vi "continous_to_binary.vi"() -> ()   [LabVIEW 2018]
uses:
  <vilib>/measure/NI_MABase.lvlib
panel:
  out "Waveform Graph 5":waveform(dbl)(graph)
  out "Waveform Graph 3":waveform(dbl)(graph)
  out "size(s)":i32
  out "Waveform Graph 2":waveform(dbl)(graph)
  in  "Fréquence":dbl(knob)=10.988369287950603 scale=0.0..100.0
  in  "Amplitude":dbl(knob)=1.3927187800734715 scale=0.0..10.0
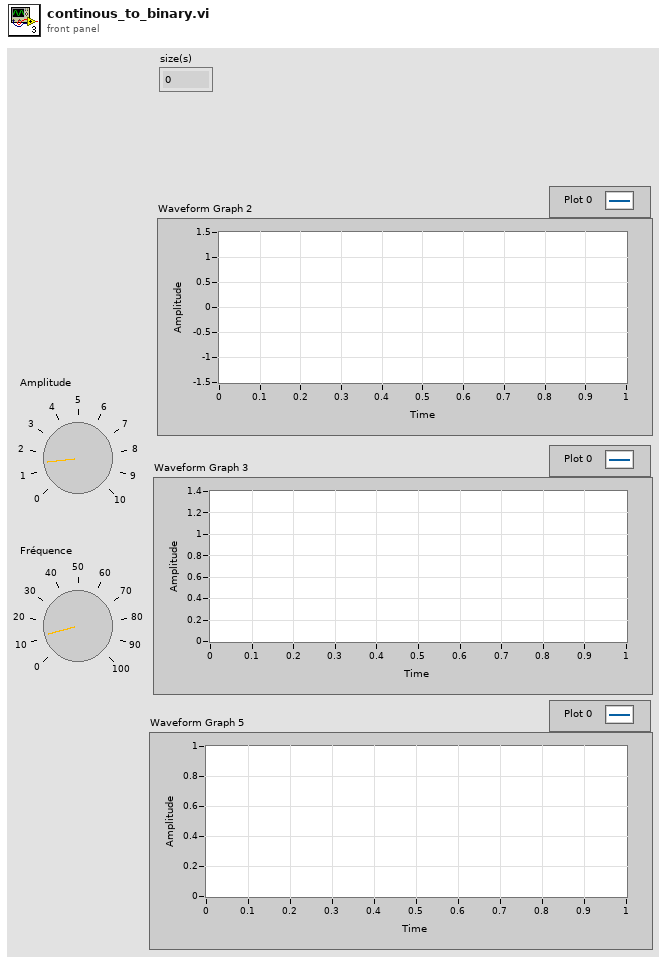
[diagram p1: front panel]
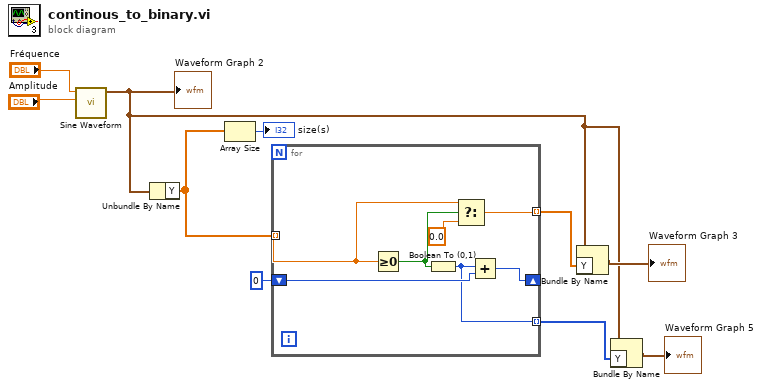
[diagram p0: block diagram]
diagram:
  n1 = call <vilib>:"Sine Waveform.vi"("amplitude"="Amplitude", "frequency"="Fréquence") -> ("signal out"=w1:waveform(dbl))  [unwired: 8 in, 1 out]
  "Waveform Graph 2" <- w1
  n2 = Unbundle By Name(w1) -> ("Y"=w6:dbl[])
  n3 = Array Size(array=w6) -> (size(s)=→"size(s)":i32)
  n4 = for {
    tunnel: w6 -> [w16] mode=indexing
    tunnel: [w12] -> w4 mode=indexing
    shift-right: [w14] -> _
    shift-left: i16 0 -> [w13]
    tunnel: [w11] -> w3 mode=indexing
    n5 = Greater Or Equal To 0?(x=w16) -> (x >= 0?=w17:bool)
    n6 = Boolean To (0,1)(Boolean=w17) -> (0, 1=w11:i16)
    n7 = Select(t=w16, s=w17, f=0.0) -> (s? t:f=w12:dbl)
    n8 = Add(x=w11, y=w13) -> (x+y=w14:i16)
  }
  n9 = Bundle By Name(cluster=w1, "Y"=w4) -> (→"Waveform Graph 3":waveform(dbl))
  n10 = Bundle By Name(cluster=w1, "Y"=w3) -> (→"Waveform Graph 5":waveform(dbl))
